vi "Dimensions.vi"(0 "Corresponding Object Points Array":dbl[][][](array[numeric])) -> (2 "k point-sets":i32, 3 "m dimensions":i32, 4 "n points in a point set":i32)   [LabVIEW 2020, in "ar.lvlib"]
uses:
  ar.lvlib
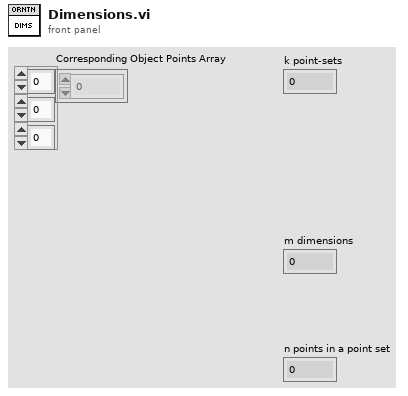
[diagram p1: front panel]
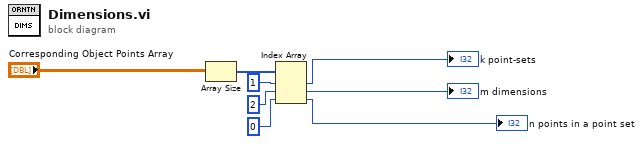
[diagram p0: block diagram]
diagram:
  n1 = Array Size(array="Corresponding Object Points Array") -> (size(s)=w2:i32[])
  n2 = Index Array(array=w2, index #1=1 ("index"), index #2=2 ("index"), index #3=0 ("index")) -> (element #1=→"k point-sets":i32, element #2=→"m dimensions":i32, element #3=→"n points in a point set":i32)
